vi "New.vi"(10 "Reseek after # bad polarizations (4)":u32=4, 11 "Number of samples (3)":i32=3) -> (0 "error out":errorcluster, 3 "Automation out":refnum<class "NMR Data.lvclass">)   [LabVIEW 2019, in "NMR Data.lvclass"]
uses:
  NMR Data.lvclass
  NMR Data.lvclass/NMR Data.ctl
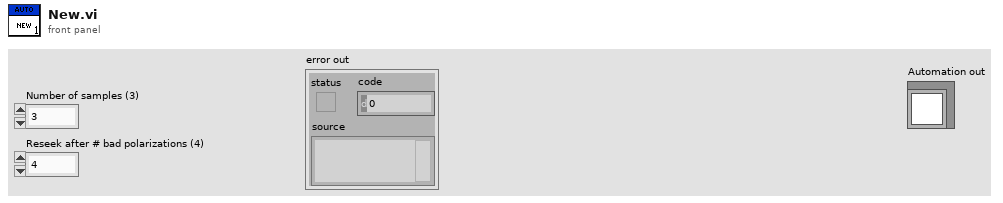
[diagram p1: front panel]
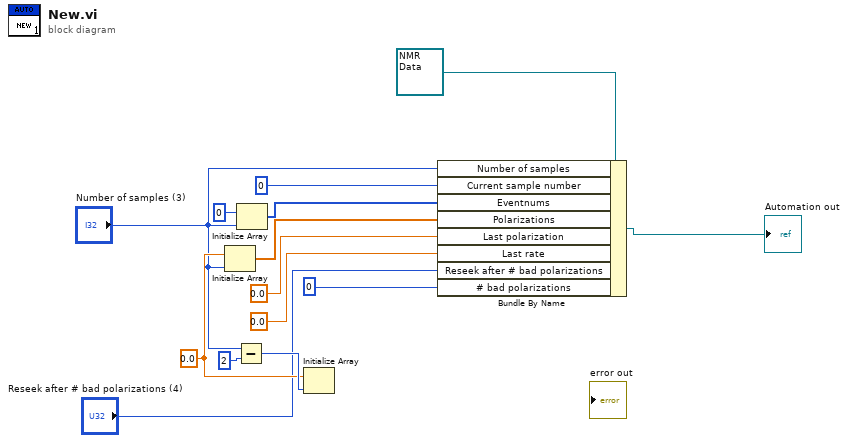
[diagram p0: block diagram]
diagram:
  w10 = 0.0 ("element")
  n1 = Initialize Array(w10, "Number of samples (3)") -> (w5:dbl[])
  n2 = Subtract(x="Number of samples (3)", y=2) -> (x-y=w12:i32)
  n3 = Initialize Array(i64 0 ("element"), "Number of samples (3)") -> (w6:i64[])
  n4 = Initialize Array(w10, w12) -> ()  [unwired: 1 out]
  n5 = Bundle By Name(cluster=refnum<class "NMR Data.lvclass"> refnum ("Automation.lvclass"), "Number of samples"="Number of samples (3)", "Current sample number"=0, "Eventnums"=w6, "Polarizations"=w5, "Last polarization"=0.0, "Last rate"=0.0, "Reseek after # bad polarizations"="Reseek after # bad polarizations (4)", "# bad polarizations"=u32 0) -> (→"Automation out":refnum<class "NMR Data.lvclass">)
